vi "helper_CCD_Setup.vi"(8 "error in":errorcluster) -> (0 "error out":errorcluster, 1 "Module Was Already Running?":bool, 2 "device open for communication?":bool, 3 "CCD out":refnum<class "CCD.lvclass">)   [LabVIEW 2023, in "horiba.test.lvlib"]
uses:
  horiba.test.lvlib
  Classes/DeviceManager/DeviceManager.lvlib
  <userlib>/_OpenG.lib/error/error.llb/openg_error.lvlib
  Classes/CCD/CCD.lvclass
panel:
  # "Connector Pane"
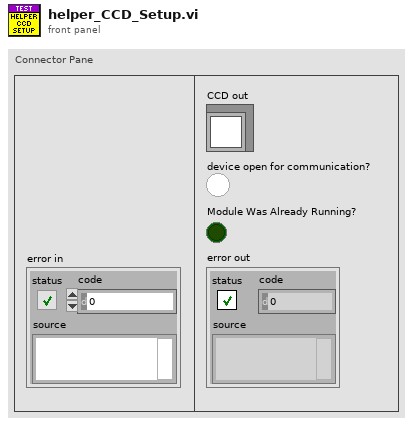
[diagram p1: front panel]
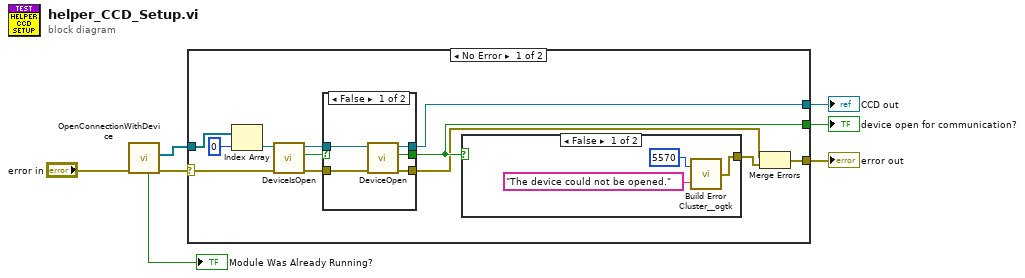
[diagram p0: block diagram]
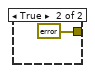
[diagram p3: hidden frame]
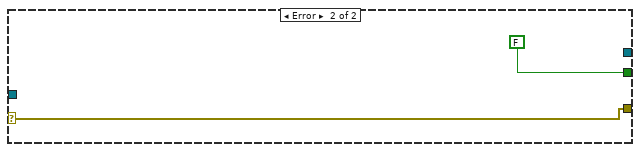
[diagram p4: hidden frame]
diagram:
  n1 = call "OpenConnectionWithDevice.vi"("error in"="error in") -> ("error out"=w4:errorcluster, "CCDs"=w2:refnum<class "CCD.lvclass">[], "Module Was Already Running?"=→"Module Was Already Running?":bool)  [unwired: 6 in, 2 out]
  n2 = case shown="No Error" w4 {
    selector: w4 -> [w11 w33]
    tunnel: w2 -> [w19 _]
    tunnel: [w17 w33] -> w6
    tunnel: [w15 FALSE ("CCD open for communication?")] -> w5
    tunnel: [w13 _] -> w1
    frame No Error {
      n3 = Index Array(array=w19, index=0) -> (element=w12:refnum<class "CCD.lvclass">)
      n4 = call-dynamic "DeviceIsOpen.vi"("error in (no error)"=w11, "CCD in"=w12) -> ("error out"=w10:errorcluster, "device is open?"=w9:bool, "CCD out"=w8:refnum<class "CCD.lvclass">)  [unwired: 6 in, 1 out]
      n5 = case shown="False" w9 {
        selector: w9 -> [_ w25]
        tunnel: [w24 w25] -> w15
        tunnel: [w23 w26] -> w14
        tunnel: [w22 w27] -> w13
        tunnel: w10 -> [w21 w26]
        tunnel: w8 -> [w20 w27]
        frame False {
          n6 = call-dynamic "DeviceOpen.vi"("error in (no error)"=w21, "CCD in"=w20) -> ("error out"=w23:errorcluster, "device is open?"=w24:bool, "CCD out"=w22:refnum<class "CCD.lvclass">)  [unwired: 6 in, 1 out]
        }
        frame True {
        }
      }
      n7 = case shown="False" w15 {
        tunnel: [w29 errorcluster {"status"=FALSE, "code"=0, "source"=""} ("error in 2")] -> w16
        frame False {
          n8 = call <userlib>:"Build Error Cluster__ogtk.vi"("String to Prepend to source (\"\")"="The device could not be opened." ("String to Prepend to source (\"\")"), "code"=5570) -> ("error out"=w29:errorcluster)
        }
        frame True {
        }
      }
      n9 = Merge Errors(w14, w16) -> (w17:errorcluster)
    }
    frame Error {
    }
  }
  "error out" <- w6
  "device open for communication?" <- w5
  "CCD out" <- w1
